vi "SetDefaultParams.vi"(8 "error in (no error)":errorcluster, 11 "Class In":refnum<class "NISTFGenPluginsBase.lvclass">) -> (0 "error out":errorcluster, 3 "Class Out":refnum<class "NISTFGenPluginsBase.lvclass">)   [LabVIEW 2014, in "FGenPlugins.lvlib" / "NISTFGenPluginsBase.lvclass"]
uses:
  NISTFGenPluginsBase.lvclass
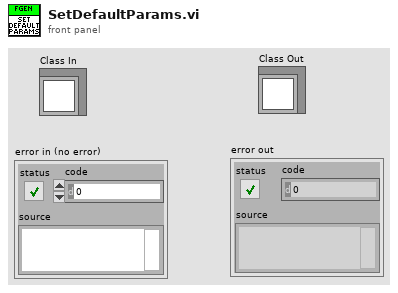
[diagram p1: front panel]
types:
  T1 = typedef "FGenPlugins.lvlib/NISTFGenPluginsBase.lvclass/ChannelParamElement.ctl" = cluster{"sName":string, "eOperateMode":u16, "bEnabled":bool, "eOutputMode":u16, "iIndex":i32, "iNameBufferSize":i32, "fGain":dbl}
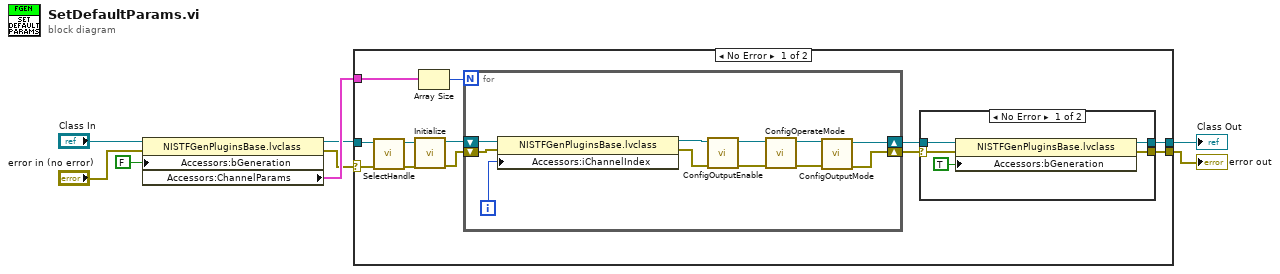
[diagram p0: block diagram]
diagram:
  n1 = property class="NISTFGenPluginsBase.lvclass"(reference="Class In", error in="error in (no error)", "Accessors:bGeneration"=FALSE ("bGeneration")) -> (reference out=w2:refnum<class "NISTFGenPluginsBase.lvclass">, error out=w1:errorcluster, "Accessors:ChannelParams"=w4:T1[])
  n2 = case shown="No Error" w1 {
    selector: w1 -> [w10 w39]
    tunnel: [w19 w40] -> w6
    tunnel: w2 -> [w12 w40]
    tunnel: w4 -> [w15 _]
    tunnel: [w14 w39] -> w3
    frame No Error {
      n3 = call-dynamic "SelectHandle.vi"("error in (no error)"=w10, "ClassIn"=w12) -> ("error out"=w9:errorcluster, "ClassOut"=w11:refnum<class "NISTFGenPluginsBase.lvclass">)  [unwired: 8 in]
      n4 = call-dynamic "Initialize.vi"("error in (no error)"=w9, "ClassIn"=w11) -> ("error out"=w17:errorcluster, "ClassOut"=w18:refnum<class "NISTFGenPluginsBase.lvclass">)  [unwired: 8 in]
      n5 = Array Size(array=w15) -> (size(s)=w16:i32)
      n6 = for {
        N: w16 -> [_]
        shift-right: [w30] -> w13
        shift-left: w17 -> [w33]
        shift-right: [w31] -> w20
        shift-left: w18 -> [w34]
        i -> [w32]
        n7 = property class="NISTFGenPluginsBase.lvclass"(reference=w34, error in=w33, "Accessors:iChannelIndex"=w32) -> (reference out=w29:refnum<class "NISTFGenPluginsBase.lvclass">, error out=w28:errorcluster)
        n8 = call-dynamic "ConfigOutputEnable.vi"("error in (no error)"=w28, "ClassIn"=w29) -> ("error out"=w37:errorcluster, "ClassOut"=w38:refnum<class "NISTFGenPluginsBase.lvclass">)  [unwired: 8 in]
        n9 = call-dynamic "ConfigOperateMode.vi"("error in (no error)"=w37, "ClassIn"=w38) -> ("error out"=w35:errorcluster, "ClassOut"=w36:refnum<class "NISTFGenPluginsBase.lvclass">)  [unwired: 8 in]
        n10 = call-dynamic "ConfigOutputMode.vi"("error in (no error)"=w35, "ClassIn"=w36) -> ("error out"=w30:errorcluster, "ClassOut"=w31:refnum<class "NISTFGenPluginsBase.lvclass">)  [unwired: 8 in]
      }
      n11 = case shown="No Error" w13 {
        selector: w13 -> [w21 w26]
        tunnel: w20 -> [w25 w27]
        tunnel: [w24 w27] -> w19
        tunnel: [w22 w26] -> w14
        frame No Error {
          n12 = property class="NISTFGenPluginsBase.lvclass"(reference=w25, error in=w21, "Accessors:bGeneration"=TRUE ("bGeneration")) -> (reference out=w24:refnum<class "NISTFGenPluginsBase.lvclass">, error out=w22:errorcluster)
        }
        frame Error {
        }
      }
    }
    frame Error {
    }
  }
  "Class Out" <- w6
  "error out" <- w3
